vi "GetFirstScreen.vi"(8 "error in (no error)":errorcluster, 11 "Bouncer in":refnum<class "Bouncer.lvclass">) -> (0 "error out":errorcluster, 2 "Array":u32[][](array[numeric]), 3 "Bouncer out":refnum<class "Bouncer.lvclass">)   [LabVIEW 2019, in "RT_Game.lvlib" / "Bouncer.lvclass"]
uses:
  Bouncer.lvclass
  Engine/Engine.lvclass
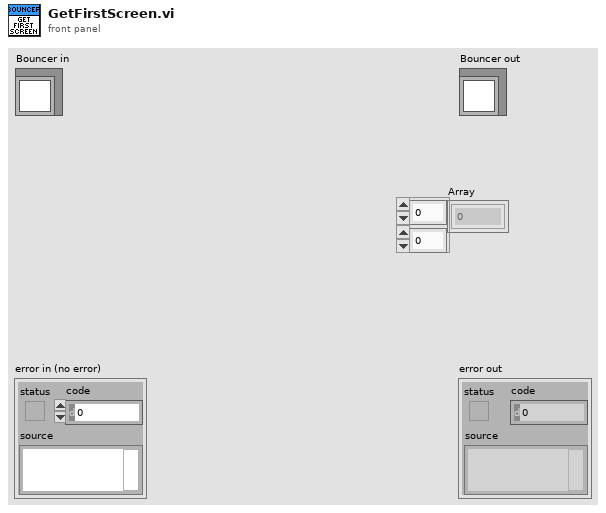
[diagram p1: front panel]
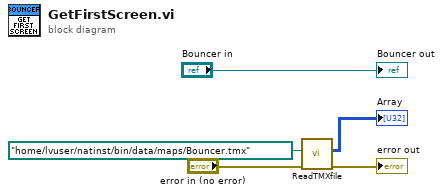
[diagram p0: block diagram]
diagram:
  n1 = call "ReadTMXfile.vi"("error in (no error)"="error in (no error)", "path to tmx-file (created with Tiles2D)"=path "/home/lvuser/natinst/bin/data/maps/Bouncer.tmx") -> ("error out"=→"error out":errorcluster, "Tilenumbers"=→"Array":u32[][])  [unwired: 8 in]
  "Bouncer out" <- "Bouncer in"
